vi "Motion Profile Generator-Optimized.vi"(0 "Max Speed (rotations/sec)":dbl, 5 "Max Acceleration (rotations/sec^2)":dbl, 7 "Max Jerk (rotations/sec^3)":dbl, 9 "Rotations to Travel":dbl, 11 "Motion Profile Control Frame Rate":dbl) -> (4 "Position rotations":dbl[](array[numeric]), 6 "velocity rotations/sec":dbl[](array[numeric]))   [LabVIEW 2016]
panel:
  out "Run Time (ms)":u32
  # "This is tempory and for testing purposes only"
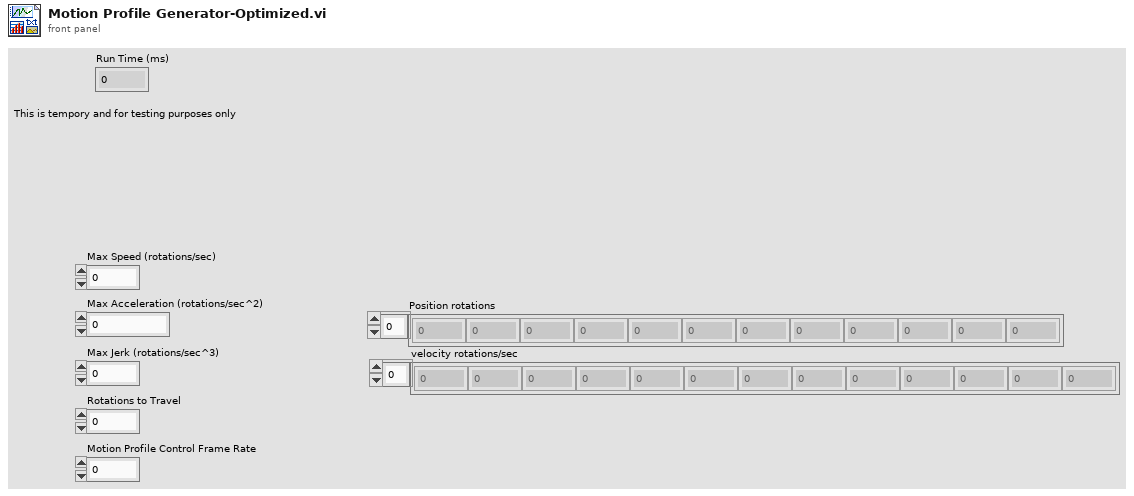
[diagram p1: front panel]
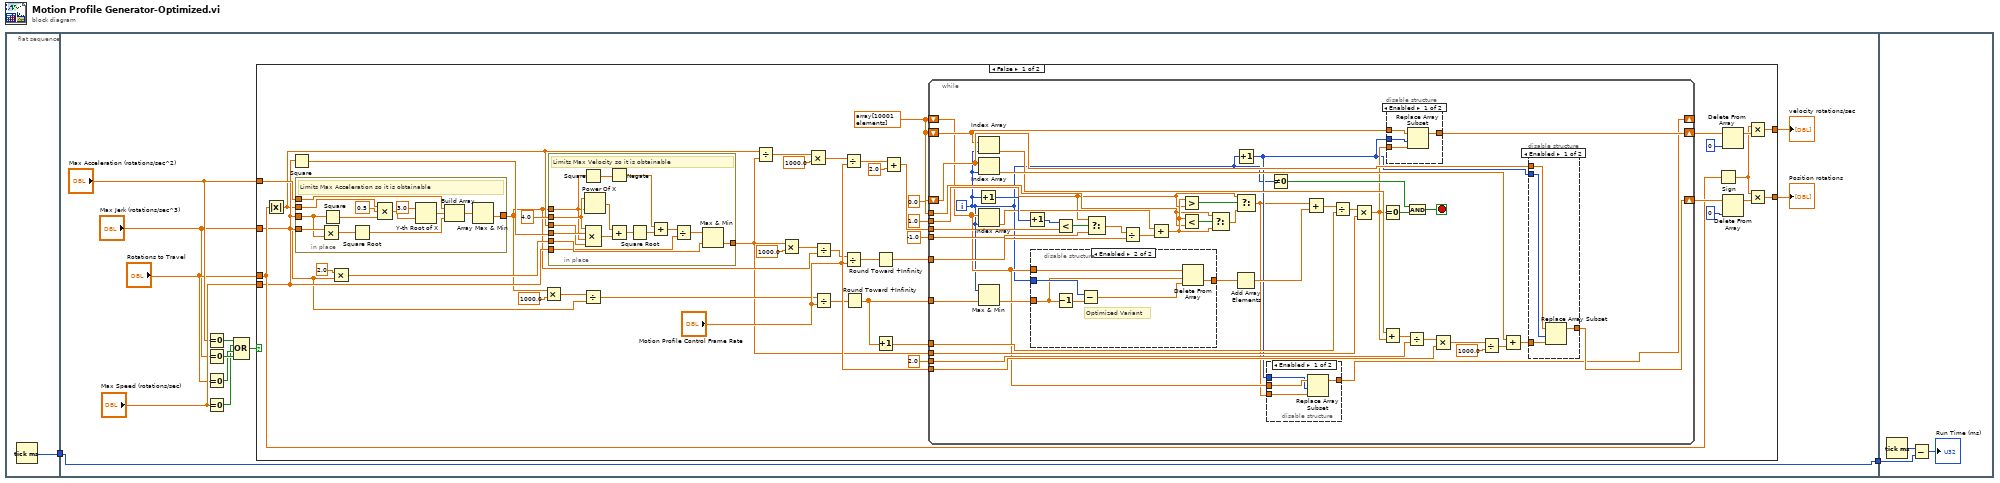
[diagram p0: block diagram]
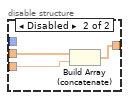
[diagram p2: hidden frame]
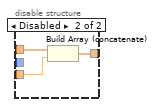
[diagram p3: hidden frame]
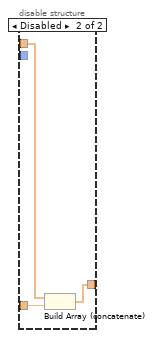
[diagram p4: hidden frame]
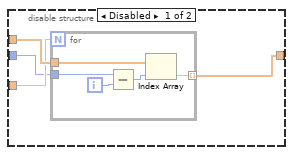
[diagram p5: hidden frame]
diagram:
  n1 = flat-sequence {
    tunnel: [w3] -> w1
    tunnel: [w4] -> w2
    tunnel: w1 -> [w4]
    tunnel: w2 -> [w169]
    frame #0 {
      n2 = Tick Count (ms)() -> (millisecond timer value=w3:u32)
    }
    frame #1 {
      n3 = Equal To 0?(x="Max Acceleration (rotations/sec^2)") -> (x = 0?=w13:bool)
      n4 = Equal To 0?(x="Max Jerk (rotations/sec^3)") -> (x = 0?=w8:bool)
      n5 = Equal To 0?(x="Rotations to Travel") -> (x = 0?=w7:bool)
      n6 = Equal To 0?(x="Max Speed (rotations/sec)") -> (x = 0?=w6:bool)
      n7 = Compound Arithmetic op=OR(w13, w6, w7, w8) -> (w5:bool)
      n8 = case shown="False" w5 {
        tunnel: "Max Acceleration (rotations/sec^2)" -> [w44 _]
        tunnel: "Max Speed (rotations/sec)" -> [w43 _]
        tunnel: "Max Jerk (rotations/sec^3)" -> [w42 _]
        tunnel: [w48 _] -> w15
        tunnel: [w47 _] -> w14
        tunnel: "Rotations to Travel" -> [w46 _]
        frame False {
          w16 = dbl[] array[10001 elements]
          n9 = Absolute Value(x=w46) -> (abs(x)=w26:dbl)
          n10 = Square(x=w42) -> (x^2=w29:dbl)
          n11 = in-place {
            in-place-border: w42 -> [w77]
            in-place-border: w44 -> [w81]
            in-place-border: [w74] -> w24
            in-place-border: w26 -> [w86]
            in-place-border: w43 -> [w78]
            # "Limits Max Acceleration so it is obtainable"
            n12 = Multiply(x=w78, y=w77) -> (x*y=w79:dbl)
            n13 = Square(x=w77) -> (x^2=w84:dbl)
            n14 = Square Root(x=w79) -> (sqrt(x)=w76:dbl)
            n15 = Compound Arithmetic op=MULTIPLY(w86, 0.5 ("value"), w84) -> (w83:dbl)
            n16 = Y-th Root of X(1:w83, 2:3.0 ("y")) -> (0:w80:dbl)
            n17 = Build Array(w81, w80, w76) -> (w75:dbl[])
            n18 = Array Max & Min(array=w75) -> (min value=w74:dbl)  [unwired: 3 out]
          }
          n19 = Multiply(x=2.0, y=w42) -> (x*y=w27:dbl)
          n20 = Multiply(x=w24, y=1000.0) -> (x*y=w25:dbl)
          n21 = in-place {
            in-place-border: w43 -> [w73]
            in-place-border: [w72] -> w21
            in-place-border: 4.0 ("x") -> [w68]
            in-place-border: w29 -> [w67]
            in-place-border: w27 -> [w61]
            in-place-border: w26 -> [w60]
            in-place-border: w24 -> [w59]
            # "Limits Max Velocity so it is obtainable"
            n22 = Square(x=w59) -> (x^2=w71:dbl)
            n23 = Power Of X(1:w59, 2:w68) -> (0:w69:dbl)
            n24 = Compound Arithmetic op=MULTIPLY(w68, w67, w59, w60) -> (w66:dbl)
            n25 = Negate(x=w71) -> (-x=w70:dbl)
            n26 = Add(x=w69, y=w66) -> (x+y=w65:dbl)
            n27 = Square Root(x=w65) -> (sqrt(x)=w64:dbl)
            n28 = Add(x=w70, y=w64) -> (x+y=w63:dbl)
            n29 = Divide(x=w63, y=w61) -> (x/y=w62:dbl)
            n30 = Max & Min(x=w62, y=w73) -> (min(x,y)=w72:dbl)  [unwired: 1 out]
          }
          n31 = Divide(x=w25, y=w42) -> (x/y=w32:dbl)
          n32 = Divide(x=w26, y=w21) -> (x/y=w18:dbl)
          n33 = Multiply(x=w21, y=1000.0) -> (x*y=w20:dbl)
          n34 = Multiply(x=w18, y=1000.0) -> (x*y=w17:dbl)
          n35 = Divide(x=w20, y=w24) -> (x/y=w34:dbl)
          n36 = Divide(x=w32, y="Motion Profile Control Frame Rate") -> (x/y=w31:dbl)
          n37 = Divide(x=w17, y="Motion Profile Control Frame Rate") -> (x/y=w36:dbl)
          n38 = Divide(x=w34, y="Motion Profile Control Frame Rate") -> (x/y=w33:dbl)
          n39 = Round Toward +Infinity(x=w31) -> (ceil(x): smallest int >= x=w56:dbl)
          n40 = Round Toward +Infinity(x=w33) -> (ceil(x): smallest int >= x=w57:dbl)
          n41 = Increment(x=w56) -> (x+1=w55:dbl)
          n42 = Add(x=w36, y=2.0) -> (x+y=w58:dbl)
          n43 = while {
            tunnel: w58 -> [w132]
            shift-right: [w93] -> _
            shift-left: w16 -> [w94]
            tunnel: w57 -> [w129]
            tunnel: w56 -> [w124]
            tunnel: w55 -> [w120]
            tunnel: w21 -> [w118]
            shift-right: [w95] -> w50
            shift-left: w16 -> [w97]
            shift-right: [w101] -> w54
            shift-left: w16 -> [w102]
            tunnel: "Motion Profile Control Frame Rate" -> [w109]
            tunnel: 1.0 ("t") -> [w98]
            tunnel: -1.0 ("f") -> [w105]
            tunnel: 0.0 ("y") -> [w104]
            tunnel: 2.0 ("y") -> [w103]
            i -> [w91]
            stop <- w111 stop-if-true
            n44 = Increment(x=w91) -> (x+1=w126:i32)
            n45 = Index Array(array=w97, index=w91) -> (element=w114:dbl)
            n46 = Index Array(array=w102, index=w91) -> (element=w115:dbl)
            n47 = Index Array(array=w94, index=w91) -> (element=w110:dbl)
            n48 = Max & Min(x=w91, y=w124) -> (min(x,y)=w123:dbl)  [unwired: 1 out]
            n49 = Increment(x=w126) -> (x+1=w127:i32)
            n50 = disable-structure shown="Enabled" {
              disable-tunnel: w94 -> [w157 w168]
              disable-tunnel: w123 -> [w156 w164]
              disable-tunnel: w91 -> [w155 w167]
              disable-tunnel: [w154 w163] -> w99
              frame Disabled {
                n51 = for {
                  N: w156 -> [_]
                  tunnel: w155 -> [w161]
                  tunnel: w157 -> [w159]
                  tunnel: [w158] -> w154 mode=indexing
                  i -> [w162]
                  n52 = Subtract(x=w161, y=w162) -> (x-y=w160:i32)
                  n53 = Index Array(array=w159, index=w160) -> (element=w158:dbl)
                }
              }
              frame Enabled {
                # "Optimized Variant"
                n54 = Decrement(x=w164) -> (x-1=w166:dbl)
                n55 = Subtract(x=w167, y=w166) -> (x-y=w165:dbl)
                n56 = Delete From Array(array=w168, length=w164, index=w165) -> (deleted portion=w163:dbl[])  [unwired: 1 out]
              }
            }
            n57 = Less?(x=w127, y=w132) -> (x < y?=w131:bool)
            n58 = Select(t=w98, s=w131, f=w105) -> (s? t:f=w130:dbl)
            n59 = Divide(x=w130, y=w129) -> (x/y=w128:dbl)
            n60 = Add(x=w110, y=w128) -> (x+y=w125:dbl)
            n61 = Greater?(x=w125, y=w98) -> (0:w89:bool)
            n62 = Less?(x=w125, y=w104) -> (x < y?=w87:bool)
            n63 = Select(t=w104, s=w87, f=w125) -> (s? t:f=w88:dbl)
            n64 = Add Array Elements(numeric array=w99) -> (sum=w122:dbl)
            n65 = Increment(x=w91) -> (x+1=w92:i32)
            n66 = Select(t=w98, s=w89, f=w88) -> (s? t:f=w90:dbl)
            n67 = disable-structure shown="Enabled" {
              disable-tunnel: w94 -> [w136 w139]
              disable-tunnel: [w135 w137] -> w93
              disable-tunnel: w92 -> [w134 _]
              disable-tunnel: w90 -> [w133 w138]
              frame Enabled {
                n68 = Replace Array Subset(array=w136, new element=w133, index=w134) -> (w135:dbl[])
              }
              frame Disabled {
                n69 = Build Array (concatenate)(w139, w138) -> (w137:dbl[])
              }
            }
            n70 = Not Equal To 0?(x=w91) -> (x != 0?=w112:bool)
            n71 = Add(x=w90, y=w122) -> (x+y=w121:dbl)
            n72 = Divide(x=w121, y=w120) -> (x/y=w119:dbl)
            n73 = Multiply(x=w119, y=w118) -> (x*y=w96:dbl)
            n74 = Equal To 0?(x=w96) -> (x = 0?=w113:bool)
            n75 = Add(x=w114, y=w96) -> (x+y=w117:dbl)
            n76 = disable-structure shown="Enabled" {
              disable-tunnel: w97 -> [w143 w146]
              disable-tunnel: [w142 w144] -> w95
              disable-tunnel: w92 -> [w141 _]
              disable-tunnel: w96 -> [w140 w145]
              frame Enabled {
                n77 = Replace Array Subset(array=w143, new element=w140, index=w141) -> (w142:dbl[])
              }
              frame Disabled {
                n78 = Build Array (concatenate)(w146, w145) -> (w144:dbl[])
              }
            }
            n79 = Divide(x=w117, y=w103) -> (x/y=w116:dbl)
            n80 = And(x=w112, y=w113) -> (x .and. y?=w111:bool)
            n81 = Multiply(x=w116, y=w109) -> (x*y=w108:dbl)
            n82 = Divide(x=w108, y=1000.0) -> (x/y=w107:dbl)
            n83 = Add(x=w115, y=w107) -> (x+y=w100:dbl)
            n84 = disable-structure shown="Enabled" {
              disable-tunnel: w102 -> [w150 w153]
              disable-tunnel: [w149 w151] -> w101
              disable-tunnel: w92 -> [w148 _]
              disable-tunnel: w100 -> [w147 w152]
              frame Enabled {
                n85 = Replace Array Subset(array=w150, new element=w147, index=w148) -> (w149:dbl[])
              }
              frame Disabled {
                n86 = Build Array (concatenate)(w153, w152) -> (w151:dbl[])
              }
            }
          }
          n87 = Sign(1:w46) -> (0:w45:dbl)
          n88 = Delete From Array(array=w50, index=0) -> (array with subset deleted=w49:dbl[])  [unwired: 1 in, 1 out]
          n89 = Delete From Array(array=w54, index=0) -> (array with subset deleted=w52:dbl[])  [unwired: 1 in, 1 out]
          n90 = Multiply(x=w45, y=w49) -> (x*y=w48:dbl[])
          n91 = Multiply(x=w45, y=w52) -> (x*y=w47:dbl[])
        }
        frame True {
        }
      }
      "velocity rotations/sec" <- w15
      "Position rotations" <- w14
    }
    frame #2 {
      n92 = Tick Count (ms)() -> (millisecond timer value=w171:u32)
      n93 = Subtract(x=w171, y=w169) -> (x-y=→"Run Time (ms)":u32)
    }
  }
